vi "Get Units.vi"(3 "Error In":errorcluster, 5 "Database Connection":refnum<k7>) -> (0 "Error Out":errorcluster, 1 "UnitNames":string[](array[string]), 2 "UnitIds":string[](array[string]))   [LabVIEW 2019]
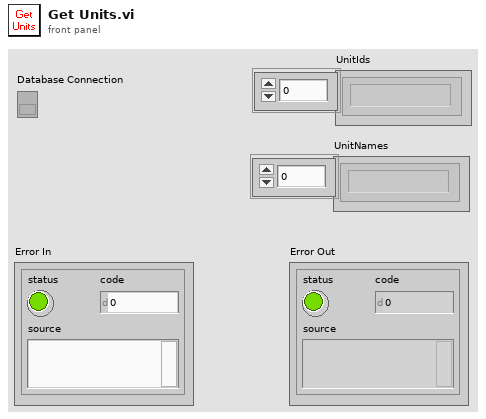
[diagram p1: front panel]
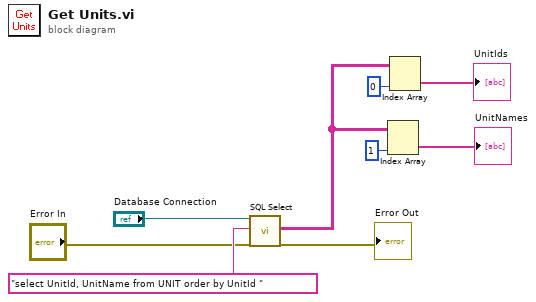
[diagram p0: block diagram]
diagram:
  n1 = call <vilib>:"SQL Select.vi"("Connection In"="Database Connection", "SQL Query"="select UnitId, UnitName from UNIT order by UnitId ", "Error in (no error)"="Error In") -> ("Data"=w2:string[][], "Error out"=→"Error Out":errorcluster)  [unwired: 14 in, 1 out]
  n2 = Index Array(array=w2, index (col)=1 ("disabled index (col)")) -> (element=→"UnitNames":string[])  [unwired: 1 in]
  n3 = Index Array(array=w2, index (col)=0 ("disabled index (col)")) -> (element=→"UnitIds":string[])  [unwired: 1 in]
